vi "BRig_Host__Loop_Consumer_RunState__typeTrial__subtypeSelResult_parse.vi"(0 "input_strCmd":string) -> (3 "output_selResult":bool, 4 "output_nTrial":u16, 6 "output_sSelection":u16, 8 "output_tSelection":u16, 10 "output_iReward_or_iError":u16, 15 "output_LorR":u16)   [LabVIEW 2014]
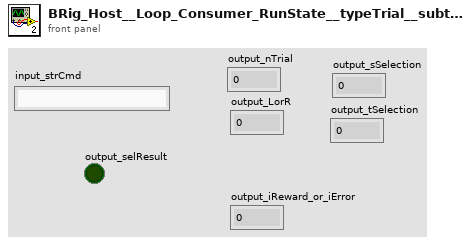
[diagram p1: front panel]
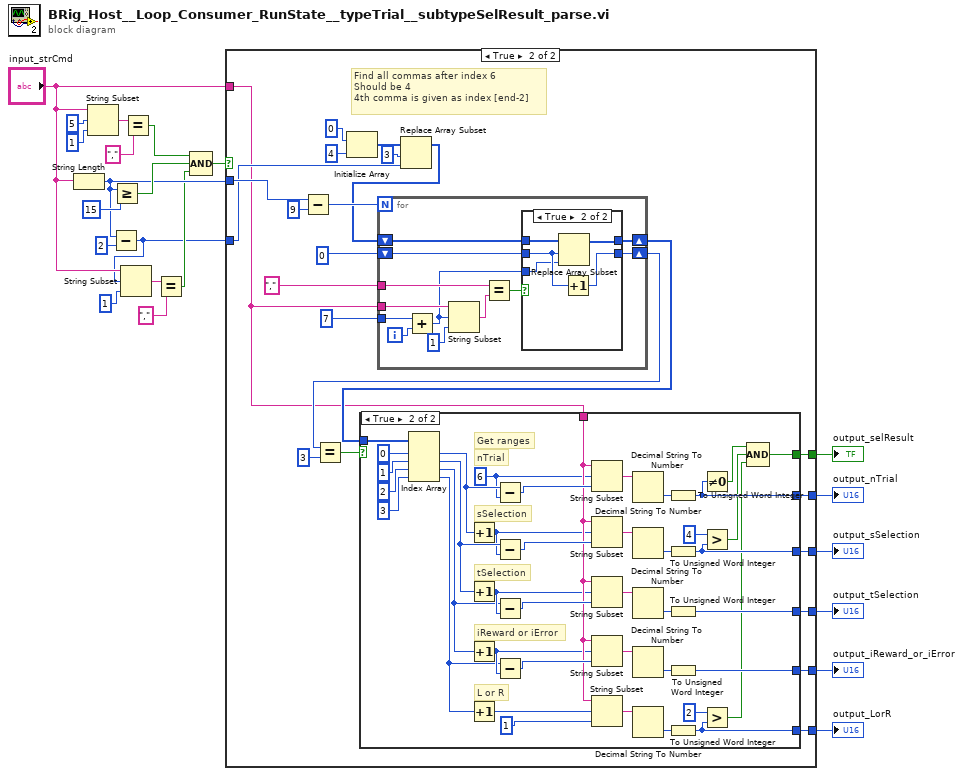
[diagram p0: block diagram]
diagram:
  n1 = String Length(string="input_strCmd") -> (length=w10:i32)
  n2 = String Subset(string="input_strCmd", offset (0)=5, length (rest)=1 ("offset (0)")) -> (substring=w20:string)
  n3 = Subtract(x=w10, y=2) -> (x-y=w7:i32)
  n4 = Greater Or Equal?(x=w10, y=15) -> (x >= y?=w17:bool)
  n5 = String Subset(string="input_strCmd", offset (0)=w7, length (rest)=1 ("offset (0)")) -> (substring=w12:string)
  n6 = Equal?(x=w20, y=",") -> (x = y?=w16:bool)
  n7 = Equal?(x=w12, y=",") -> (x = y?=w8:bool)
  n8 = Compound Arithmetic op=AND(w16, w17, w8) -> (w15:bool)
  n9 = case shown="True" w15 {
    tunnel: "input_strCmd" -> [_ w30]
    tunnel: w10 -> [_ w42]
    tunnel: w7 -> [_ w33]
    tunnel: [_ w28] -> w6
    tunnel: [_ w27] -> w5
    tunnel: [_ w26] -> w4
    tunnel: [_ w25] -> w3
    tunnel: [_ w24] -> w2
    tunnel: [_ w23] -> w1
    frame False {
    }
    frame True {
      # "Find all commas after index 6\nShould be 4\n4th comma is given as index [end-2]"
      n10 = Subtract(x=w42, y=9) -> (x-y=w41:i32)
      n11 = Initialize Array(0 ("element"), 4 ("dimension size")) -> (w35:i32[])
      n12 = Replace Array Subset(array=w35, new element=w33, index=3) -> (w34:i32[])
      n13 = for {
        N: w41 -> [_]
        tunnel: w30 -> [w97]
        tunnel: "," ("y") -> [w95]
        tunnel: 7 ("element") -> [w93]
        shift-right: [w87] -> w37
        shift-left: 0 ("element") -> [w89]
        shift-right: [w88] -> w31
        shift-left: w34 -> [w90]
        i -> [w94]
        n14 = Add(x=w93, y=w94) -> (x+y=w91:i32)
        n15 = String Subset(string=w97, offset (0)=w91, length (rest)=1 ("offset (0)")) -> (substring=w96:string)
        n16 = Equal?(x=w95, y=w96) -> (x = y?=w92:bool)
        n17 = case shown="True" w92 {
          tunnel: w91 -> [_ w102]
          tunnel: w90 -> [w100 w105]
          tunnel: w89 -> [w99 w103]
          tunnel: [w100 w104] -> w88
          tunnel: [w99 w101] -> w87
          frame False {
          }
          frame True {
            n18 = Replace Array Subset(array=w105, new element=w102, index=w103) -> (w104:i32[])
            n19 = Increment(x=w103) -> (x+1=w101:i32)
          }
        }
      }
      n20 = Equal?(x=w37, y=3) -> (x = y?=w29:bool)
      n21 = case shown="True" w29 {
        tunnel: w31 -> [_ w86]
        tunnel: w30 -> [_ w77]
        tunnel: [_ w54] -> w28
        tunnel: [_ w50] -> w27
        tunnel: [_ w53] -> w26
        tunnel: [_ w64] -> w25
        tunnel: [_ w63] -> w24
        tunnel: [_ w46] -> w23
        frame False {
        }
        frame True {
          w61 = 6 ("y")
          # "L or R"
          # "iReward or iError"
          # "tSelection"
          # "sSelection"
          # "nTrial"
          # "Get ranges"
          n22 = Index Array(array=w86, index #1=0 ("index"), index #2=1 ("index"), index #3=2 ("index"), index #4=3 ("index")) -> (element #1=w62:i32, element #2=w60:i32, element #3=w55:i32, element #4=w57:i32)
          n23 = Increment(x=w62) -> (x+1=w59:i32)
          n24 = Increment(x=w60) -> (x+1=w56:i32)
          n25 = Increment(x=w55) -> (x+1=w58:i32)
          n26 = Increment(x=w57) -> (x+1=w76:i32)
          n27 = Subtract(x=w62, y=w61) -> (x-y=w81:i32)
          n28 = Subtract(x=w60, y=w59) -> (x-y=w80:i32)
          n29 = Subtract(x=w55, y=w56) -> (x-y=w79:i32)
          n30 = Subtract(x=w57, y=w58) -> (x-y=w78:i32)
          n31 = String Subset(string=w77, offset (0)=w61, length (rest)=w81) -> (substring=w74:string)
          n32 = String Subset(string=w77, offset (0)=w59, length (rest)=w80) -> (substring=w73:string)
          n33 = String Subset(string=w77, offset (0)=w56, length (rest)=w79) -> (substring=w72:string)
          n34 = String Subset(string=w77, offset (0)=w58, length (rest)=w78) -> (substring=w71:string)
          n35 = String Subset(string=w77, offset (0)=w76, length (rest)=1 ("y")) -> (substring=w70:string)
          n36 = Decimal String To Number(string=w74) -> (number=w69:i32)  [unwired: 2 in, 1 out]
          n37 = Decimal String To Number(string=w73) -> (number=w68:i32)  [unwired: 2 in, 1 out]
          n38 = Decimal String To Number(string=w72) -> (number=w67:i32)  [unwired: 2 in, 1 out]
          n39 = Decimal String To Number(string=w71) -> (number=w66:i32)  [unwired: 2 in, 1 out]
          n40 = Decimal String To Number(string=w70) -> (number=w65:i32)  [unwired: 2 in, 1 out]
          n41 = To Unsigned Word Integer(number=w69) -> (unsigned 16bit integer=w54:u16)
          n42 = To Unsigned Word Integer(number=w68) -> (unsigned 16bit integer=w53:u16)
          n43 = To Unsigned Word Integer(number=w67) -> (unsigned 16bit integer=w64:u16)
          n44 = To Unsigned Word Integer(number=w66) -> (unsigned 16bit integer=w63:u16)
          n45 = To Unsigned Word Integer(number=w65) -> (unsigned 16bit integer=w50:u16)
          n46 = Not Equal To 0?(x=w54) -> (x != 0?=w47:bool)
          n47 = Greater?(x=u16 4, y=w53) -> (0:w48:bool)
          n48 = Greater?(x=u16 2, y=w50) -> (0:w49:bool)
          n49 = Compound Arithmetic op=AND(w47, w48, w49) -> (w46:bool)
        }
      }
    }
  }
  "output_nTrial" <- w6
  "output_LorR" <- w5
  "output_selResult" <- w1
  "output_sSelection" <- w4
  "output_tSelection" <- w3
  "output_iReward_or_iError" <- w2
